vi "Filter Data For Graph.vi"(0 "Input State":T2=[{"Base Directory"=path "", "Experimental Data"={"Experimental Data"={"Extension (nm)"=[], "Force (pN)"=[], "Name"=""}, "Enabled"=FALSE}, "Chain Fit"={"Experimental Data"={"Extension (nm)"=[], "Force (pN)"=[], "Name"=""}, "Enabled"=FALSE}, "Selected"=FALSE, "Ramp Rate (nm/s)"=0.0, "Spring Constant (pN/nm)"=0.0, "Slope (nm/V)"=0.0}]) -> (1 "Graph Entries":T1(array[cluster]), 2 "Legend Entries":string[](array[string]))   [LabVIEW 2013]
uses:
  Analysis Data.ctl
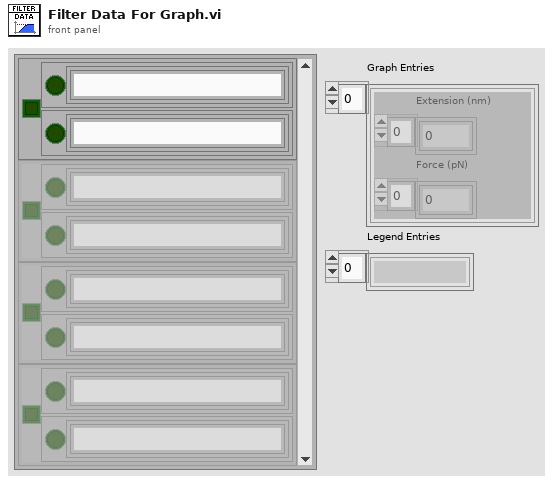
[diagram p1: front panel]
types:
  T1 = cluster{"Extension (nm)":dbl[], "Force (pN)":dbl[]}[]
  T2 = typedef "Analysis Data.ctl" = cluster{"Base Directory":path, "Experimental Data":cluster{"Experimental Data":cluster{"Extension (nm)":dbl[], "Force (pN)":dbl[], "Name":string}, "Enabled":bool}, "Chain Fit":cluster{"Experimental Data":cluster{"Extension (nm)":dbl[], "Force (pN)":dbl[], "Name":string}, "Enabled":bool}, "Selected":bool, "Ramp Rate (nm/s)":dbl, "Spring Constant (pN/nm)":dbl, "Slope (nm/V)":dbl}[]
  T3 = cluster{"Experimental Data":cluster{"Extension (nm)":dbl[], "Force (pN)":dbl[], "Name":string}, "Enabled":bool}
  T4 = cluster{"Experimental Data":cluster{"Extension (nm)":dbl[], "Force (pN)":dbl[], "Name":string}, "Enabled":bool}[]
  T5 = cluster{"Extension (nm)":dbl[], "Force (pN)":dbl[], "Name":string}
  T6 = cluster{"Extension (nm)":dbl[], "Force (pN)":dbl[]}
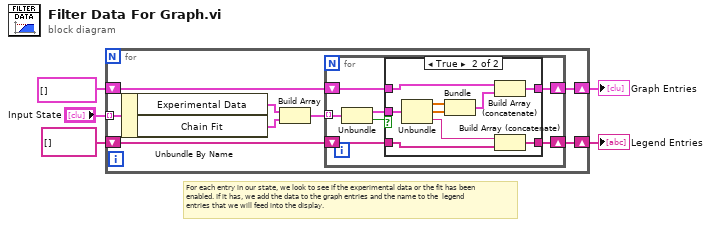
[diagram p0: block diagram]
diagram:
  # "For each entry in our state, we look to see if the experimental data or the fit has been\nenabled. If it has, we add the data to the graph entries and the name to the  legend\nentries that we will feed into the display."
  n1 = for {
    tunnel: "Input State" -> [w8] mode=indexing
    shift-right: [w11] -> w4
    shift-left: T1 [] -> [w12]
    shift-right: [w9] -> w3
    shift-left: string[] [] -> [w10]
    n2 = Unbundle By Name(w8) -> ("Experimental Data"=w7:T3, "Chain Fit"=w6:T3)
    n3 = Build Array(w7, w6) -> (w13:T4)
    n4 = for {
      tunnel: w13 -> [w20] mode=indexing
      shift-right: [w17] -> w9
      shift-left: w10 -> [w16]
      shift-right: [w15] -> w11
      shift-left: w12 -> [w14]
      n5 = Unbundle(w20) -> ("Experimental Data"=w18:T5, "Enabled"=w19:bool)
      n6 = case shown="True" w19 {
        tunnel: w18 -> [_ w31]
        tunnel: [w22 w27] -> w17
        tunnel: w16 -> [w22 w26]
        tunnel: [w21 w24] -> w15
        tunnel: w14 -> [w21 w23]
        frame False {
        }
        frame True {
          n7 = Unbundle(w31) -> ("Extension (nm)"=w30:dbl[], "Force (pN)"=w29:dbl[], "Name"=w28:string)
          n8 = Bundle("Extension (nm)"=w30, "Force (pN)"=w29) -> (w25:T6)  [unwired: 1 in]
          n9 = Build Array (concatenate)(w23, w25) -> (w24:T1)
          n10 = Build Array (concatenate)(w28, w26) -> (w27:string[])
        }
      }
    }
  }
  "Graph Entries" <- w4
  "Legend Entries" <- w3
